vi "Determine Wheel State.vi"(8 "Allowable Variation from Ideal":dbl, 9 "Ideal Slip Percent":dbl, 10 "Chassis Speed":dbl, 11 "Wheel Speed":dbl) -> (1 "Error":dbl, 2 "Inline Slip":bool)   [LabVIEW 2015]
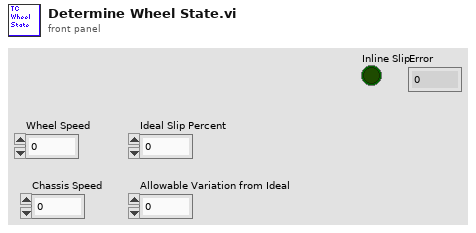
[diagram p1: front panel]
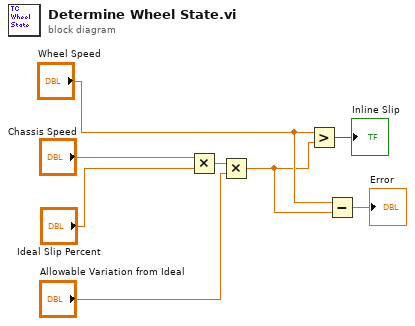
[diagram p0: block diagram]
diagram:
  n1 = Multiply(x="Chassis Speed", y="Ideal Slip Percent") -> (x*y=w6:dbl)
  n2 = Multiply(x=w6, y="Allowable Variation from Ideal") -> (x*y=w2:dbl)
  n3 = Greater?(x="Wheel Speed", y=w2) -> (0:→"Inline Slip":bool)
  n4 = Subtract(x="Wheel Speed", y=w2) -> (x-y=→"Error":dbl)
